vi "doOperation.vi"(8 "error in (no error)":errorcluster, 9 "num2":dbl, 10 "num1":dbl, 11 "OperationAdd in":refnum<class "OperationAdd.lvclass">) -> (0 "error out":errorcluster, 3 "OperationAdd out":refnum<class "OperationAdd.lvclass">)   [LabVIEW 2018, in "OperationAdd.lvclass"]
uses:
  OperationAdd.lvclass
  ConsoleOut/Print Options.ctl
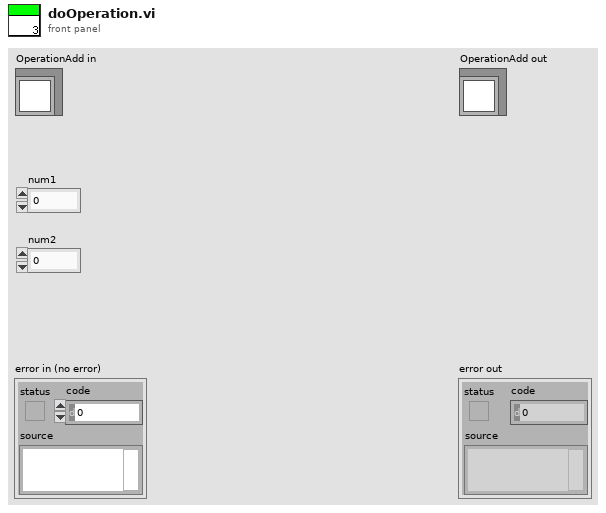
[diagram p1: front panel]
types:
  T1 = typedef "Print Options.ctl" = enum16{"Create", "Get Reference", "Print", "Print Header", "Close"}
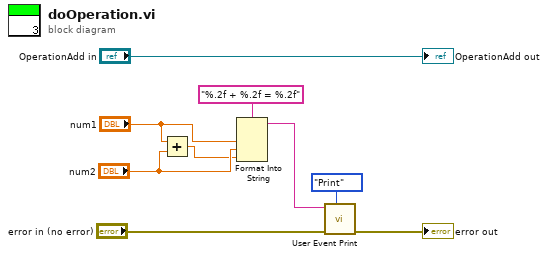
[diagram p0: block diagram]
diagram:
  n1 = Add(x="num1", y="num2") -> (x+y=w4:dbl)
  n2 = Format Into String(format string="%.2f + %.2f = %.2f", "num1", "num2", w4) -> (resulting string=w1:string)  [unwired: 2 in, 1 out]
  n3 = call "User Event Print.vi"("Options"=Print_Options."Print", "error in (no error)"="error in (no error)", "String to Print"=w1) -> ("error out"=→"error out":errorcluster)  [unwired: 7 in, 1 out]
  "OperationAdd out" <- "OperationAdd in"
